vi "Version1.0.vi"() -> ()   [LabVIEW 2012]
panel:
  in  "Initial Folder Path:":path
  in  "选项卡控件":T1(tab)
  in  "Double:":dbl
  in  "String:":string
  in  "Other:":string
  in  "Save This Shot":bool
  out "Shots:":i32
  in  "Save This Notes":bool
  in  "Other Notes:":string
  in  "Options":u16(ring) caption="Choose File:" items=["2014-5-5-Notes.txt", "2014-5-5.txt"]
  in  "查询":bool
  out "Notes:":string
  out "Shots:":i32
  out "Shot's situation:":string
  in  "Function 5":i8(knob) scale=0.0..4.0
  in  "Function 1":bool
  in  "Function 2":bool
  in  "Function 3":bool
  in  "Function 4":bool
  in  "AVT SDK Demon":bool
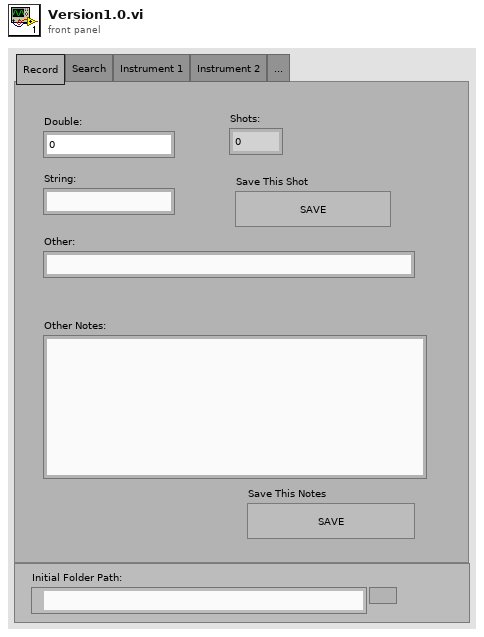
[diagram p1: front panel]
types:
  T1 = enum32{"Record", "Search", "Instrument 1", "Instrument 2", "..."}
  T2 = enum16{"open", "replace", "create", "open or create", "replace or create", "replace or create with confirmation"}
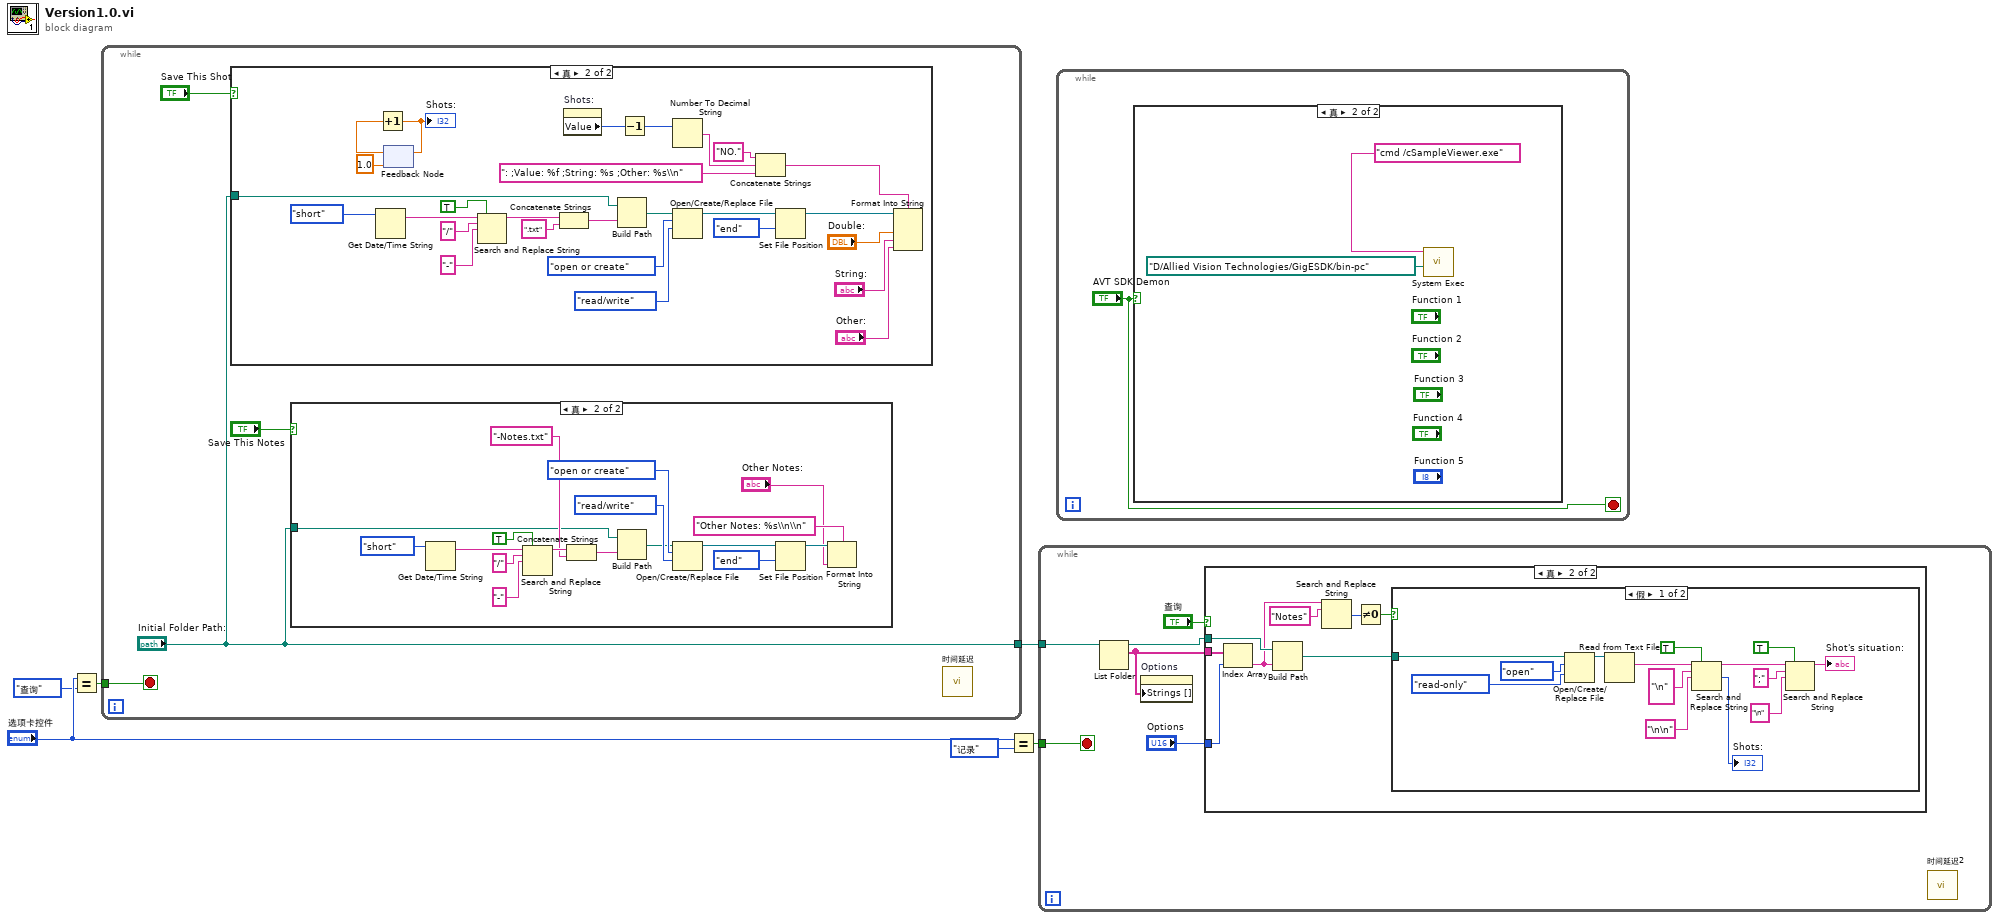
[diagram p0: block diagram]
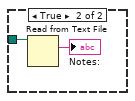
[diagram p4: hidden frame]
diagram:
  n1 = Equal?(x="选项卡控件", y=enum32{"记录", "查询"}."查询") -> (x = y?=w2:bool)
  n2 = while {
    tunnel: ["Initial Folder Path:"] -> w6
    tunnel: w2 -> [w7]
    stop <- w7 stop-if-true
    n3 = case shown="真" "Save This Shot" {
      tunnel: "Initial Folder Path:" -> [_ w34]
      frame False {
      }
      frame True {
        n4 = Get Date/Time String(date format (0)=enum16{"short", "long", "abbreviated"}."short" ("日期格式(0)")) -> (date string=w48:string)  [unwired: 2 in, 1 out]
        n5 = feedback #1(1.0 ("x")) -> (w37:dbl)
        n6 = Increment(x=w37) -> (x+1=w35:dbl)
        "Shots:" <- w35
        n7 = feedback-in #1(w35) -> ()
        n8 = Search and Replace String(replace all?=TRUE ("替换全部？(F)"), input string=w48, search string="/" ("搜索字符串"), replace string="-" ("替换字符串(\"\")")) -> (result string=w45:string)  [unwired: 4 in, 3 out]
        n9 = Concatenate Strings(w45, ".txt" ("字符串")) -> (w50:string)
        n10 = property on="Shots:" class="DigNum (严格)"() -> ("Value"=w29:i32)  [unwired: 2 in, 2 out]
        n11 = Build Path(base path=w34, name or relative path=w50) -> (appended path=w51:path)
        n12 = Decrement(x=w29) -> (x-1=w28:i32)
        n13 = Number To Decimal String(number=w28) -> (decimal integer string=w33:string)  [unwired: 1 in]
        n14 = Open/Create/Replace File(file path (use dialog)=w51, operation (0:open)=T2."open or create" ("操作(0:open)"), access (0:read/write)=enum16{"read/write", "read-only", "write-only"}."read/write" ("权限(0:read/write)")) -> (refnum out=w39:refnum<file>)  [unwired: 3 in, 2 out]
        n15 = Concatenate Strings("NO." ("字符串"), w33, ": ;Value: %f ;String: %s ;Other: %s\\n" ("格式字符串")) -> (w30:string)
        n16 = Set File Position(refnum=w39, from (0:start)=enum16{"start", "end", "current"}."end" ("自（0:起始）")) -> (refnum out=w38:refnum<file>)  [unwired: 2 in, 1 out]
        n17 = Format Into String(format string=w30, initial string=w38, "Double:", "String:", "Other:") -> ()  [unwired: 1 in, 2 out]
      }
    }
    n18 = case shown="真" "Save This Notes" {
      tunnel: "Initial Folder Path:" -> [_ w11]
      frame False {
      }
      frame True {
        n19 = Get Date/Time String(date format (0)=enum16{"short", "long", "abbreviated"}."short" ("日期格式(0)")) -> (date string=w23:string)  [unwired: 2 in, 1 out]
        n20 = Search and Replace String(replace all?=TRUE ("替换全部？(F)"), input string=w23, search string="/" ("搜索字符串"), replace string="-" ("替换字符串(\"\")")) -> (result string=w14:string)  [unwired: 4 in, 3 out]
        n21 = Concatenate Strings(w14, "-Notes.txt" ("字符串")) -> (w12:string)
        n22 = Build Path(base path=w11, name or relative path=w12) -> (appended path=w24:path)
        n23 = Open/Create/Replace File(file path (use dialog)=w24, operation (0:open)=T2."open or create" ("操作(0:open)"), access (0:read/write)=enum16{"read/write", "read-only", "write-only"}."read/write" ("权限(0:read/write)")) -> (refnum out=w17:refnum<file>)  [unwired: 3 in, 2 out]
        n24 = Set File Position(refnum=w17, from (0:start)=enum16{"start", "end", "current"}."end" ("自（0:起始）")) -> (refnum out=w16:refnum<file>)  [unwired: 2 in, 1 out]
        n25 = Format Into String(format string="Other Notes: %s\\n\\n" ("格式字符串"), initial string=w16, "Other Notes:") -> ()  [unwired: 1 in, 2 out]
      }
    }
    n26 = call "时间延迟"() -> ()  [unwired: 11 in, 1 out]
  }
  n27 = Equal?(x="选项卡控件", y=enum32{"记录", "查询"}."记录") -> (x = y?=w1:bool)
  n28 = while {
    tunnel: w6 -> [w60]
    tunnel: w1 -> [w55]
    stop <- w55 stop-if-true
    n29 = List Folder(path=w60) -> (path out=w57:path, filenames=w59:string[])  [unwired: 3 in, 2 out]
    n30 = property on="Options" class="Ring (严格)"("Strings []"=w59) -> ()  [unwired: 2 in, 2 out]
    n31 = case shown="真" "查询" {
      tunnel: w59 -> [_ w68]
      tunnel: "Options" -> [_ w67]
      tunnel: w57 -> [_ w66]
      frame False {
      }
      frame True {
        n32 = Index Array(array=w68, index=w67) -> (element=w65:string)
        n33 = Build Path(base path=w66, name or relative path=w65) -> (appended path=w61:path)
        n34 = Search and Replace String(input string=w65, search string="Notes" ("搜索字符串")) -> (number of replacements=w63:i32)  [unwired: 6 in, 3 out]
        n35 = Not Equal To 0?(x=w63) -> (x != 0?=w62:bool)
        n36 = case shown="假" w62 {
          tunnel: w61 -> [w82 w84]
          frame False {
            n37 = Open/Create/Replace File(file path (use dialog)=w82, operation (0:open)=T2."open" ("操作(0:open)"), access (0:read/write)=enum16{"read/write", "read-only", "write-only"}."read-only" ("权限(0:read/write)")) -> (refnum out=w79:refnum<file>)  [unwired: 3 in, 2 out]
            n38 = Read from Text File(file (use dialog)=w79) -> (text=w75:string)  [unwired: 3 in, 3 out]
            n39 = Search and Replace String(replace all?=TRUE ("替换全部？(F)"), input string=w75, search string="\n" ("搜索字符串"), replace string="\n\n" ("替换字符串(\"\")")) -> (result string=w72:string, number of replacements=→"Shots:":i32)  [unwired: 4 in, 2 out]
            n40 = Search and Replace String(replace all?=TRUE ("替换全部？(F)"), input string=w72, search string=";" ("搜索字符串"), replace string="\n" ("替换字符串(\"\")")) -> (result string=→"Shot's situation:":string)  [unwired: 4 in, 3 out]
          }
          frame True {
            n41 = Read from Text File(file (use dialog)=w84) -> (text=→"Notes:":string)  [unwired: 3 in, 3 out]
          }
        }
      }
    }
    n42 = call "时间延迟2"() -> ()  [unwired: 11 in, 1 out]
  }
  n43 = while {
    stop <- "AVT SDK Demon" stop-if-true
    n44 = case shown="真" "AVT SDK Demon" {
      frame False {
      }
      frame True {
        n45 = call <vilib>:"System Exec.vi"("working directory"=path "D:/Allied Vision Technologies/GigESDK/bin-pc", "command line"="cmd /cSampleViewer.exe") -> ()  [unwired: 6 in, 4 out]
      }
    }
  }
